vi "aboutDialog.vi"() -> (3 "Cancelled?":bool)   [LabVIEW 2015]
doc: "About dialog window."
uses:
  <vilib>/Platform/browser.llb/Open URL in Default Browser (string).vi
panel:
  out "exe path":path
  in  "linktausand":bool
  out "exe ver":string
  in  "OK":bool
  # "Tausand Abacus AB1004 :: Acquisition example\nExample of a complete acquisition system using a Tausand Abacus\nBuilt in LabVIEW 2015."
  # "Visit us at:"
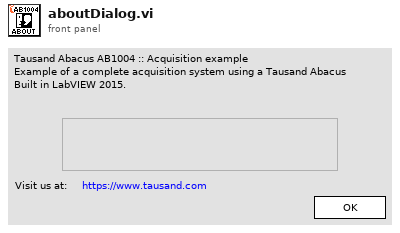
[diagram p1: front panel]
types:
  T1 = cluster{"FileVersion":string, "FileMajorPart":i32, "FileMinorPart":i32, "FileBuildPart":i32, "FilePrivatePart":i32, "Language":string, "LegalCopyright":string, "FileDescription":string, "CompanyName":string, "ProductName":string, "InternalName":string}
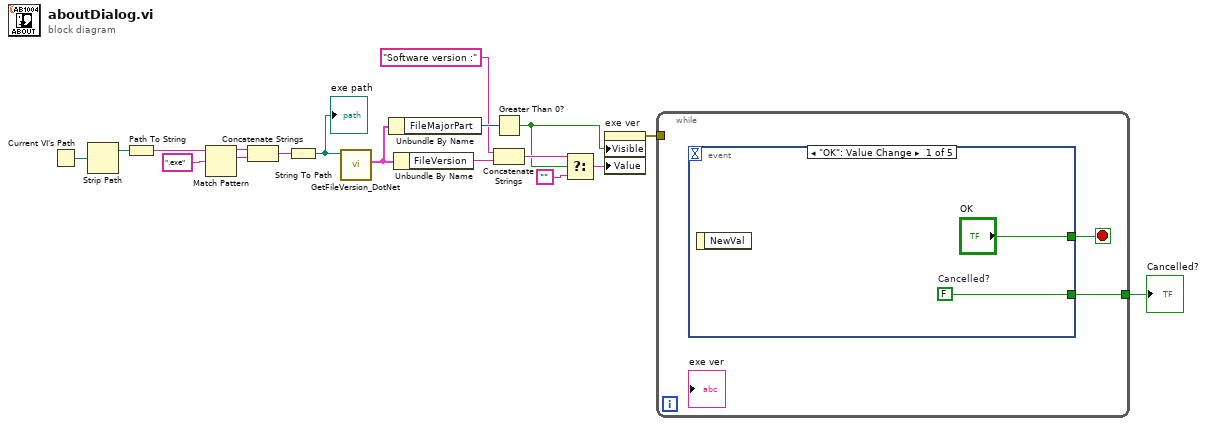
[diagram p0: block diagram]
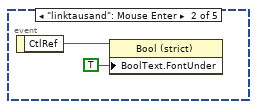
[diagram p2: hidden frame]
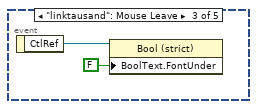
[diagram p3: hidden frame]
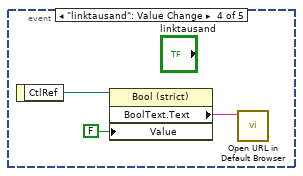
[diagram p4: hidden frame]
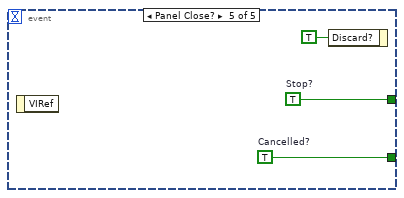
[diagram p5: hidden frame]
diagram:
  n1 = Current VI's Path() -> (path=w7:path)
  n2 = Strip Path(path=w7) -> (stripped path=w6:path)  [unwired: 1 out]
  n3 = Path To String(path=w6) -> (string=w9:string)
  n4 = Match Pattern(string=w9, regular expression=".exe") -> (before substring=w5:string, match substring=w4:string)  [unwired: 1 in, 2 out]
  n5 = Concatenate Strings(w5, w4) -> (w3:string)
  n6 = String To Path(string=w3) -> (path=w2:path)
  "exe path" <- w2
  n7 = call <instrlib>:"GetFileVersion_DotNet.vi"("Exe Path"=w2) -> ("File Info Out"=w16:T1)  [unwired: 8 in, 2 out]
  n8 = Unbundle By Name(w16) -> ("FileMajorPart"=w17:i32)
  n9 = Unbundle By Name(w16) -> ("FileVersion"=w14:string)
  n10 = Greater Than 0?(x=w17) -> (x > 0?=w1:bool)
  n11 = Concatenate Strings("Software version :" ("string"), w14) -> (w12:string)
  n12 = Select(t=w12, s=w1, f="") -> (s? t:f=w10:string)
  n13 = property on="exe ver" class="Str"("Visible"=w1, "Value"=w10) -> (error out=w11:errorcluster)  [unwired: 2 in, 1 out]
  n14 = while {
    tunnel: [w19] -> w18
    tunnel: w11 -> [_]
    stop <- w20 stop-if-true
    n15 = event shown="[0] \"OK\": Value Change" {
      selector: _ -> [_ _ _ _ _]
      dyn-events: _ -> [_ _ _ _ _]
      timeout: _ -> [_ _ _ _ _]
      tunnel: ["OK" _ _ _ w31] -> w20
      tunnel: [w22 _ _ _ w30] -> w19
      event "OK": Value Change {
        w22 = FALSE  # Cancelled?
        n16 = event-data() -> ()  [unwired: 1 in, 1 out]
      }
      event "linktausand": Mouse Enter {
        n17 = event-data() -> ("CtlRef"=w24:refnum<vi>)  [unwired: 1 in]
        n18 = property class="Bool (strict)"(reference=w24, "BoolText.FontUnder"=TRUE ("Boolean Text.Enable Hyperlinks")) -> ()  [unwired: 1 in, 2 out]
      }
      event "linktausand": Mouse Leave {
        n19 = event-data() -> ("CtlRef"=w25:refnum<vi>)  [unwired: 1 in]
        n20 = property class="Bool (strict)"(reference=w25, "BoolText.FontUnder"=FALSE ("Boolean Text.Enable Hyperlinks")) -> ()  [unwired: 1 in, 2 out]
      }
      event "linktausand": Value Change {
        n21 = event-data() -> ("CtlRef"=w29:refnum<vi>)  [unwired: 1 in]
        n22 = property class="Bool (strict)"(reference=w29, "Value"=FALSE) -> ("BoolText.Text"=w28:string)  [unwired: 1 in, 2 out]
        n23 = call-poly <vilib>:"Open URL in Default Browser.vi"("URL"=w28) -> ()  [unwired: 5 in, 2 out]
      }
      event Panel Close? {
        w30 = TRUE  # Cancelled?
        w31 = TRUE  # Stop?
        n24 = event-data() -> ()  [unwired: 1 in, 1 out]
        n25 = event-data("Discard?"=TRUE) -> ()  [unwired: 1 in, 1 out]
      }
    }
  }
  "Cancelled?" <- w18
